vi "Adv_Close_Image.vi"(8 "error in (no error)":errorcluster, 10 "ImageDataSet":refnum<k24>, 11 "LightField Automation in":refnum<class "LightField Automation.lvclass">) -> (0 "error out":errorcluster, 3 "LightField Automation out":refnum<class "LightField Automation.lvclass">)   [LabVIEW 2015, in "LightField Automation.lvclass"]
uses:
  LightField Automation.lvclass
  C:/Program Files/Princeton Instruments/LightField/AddInViews/PrincetonInstruments.LightFieldViewV3.dll
  Program Files/Princeton Instruments/LightField/AddInViews/PrincetonInstruments.LightFieldViewV3.dll
  LightField Automation.lvclass/LightField Automation.ctl
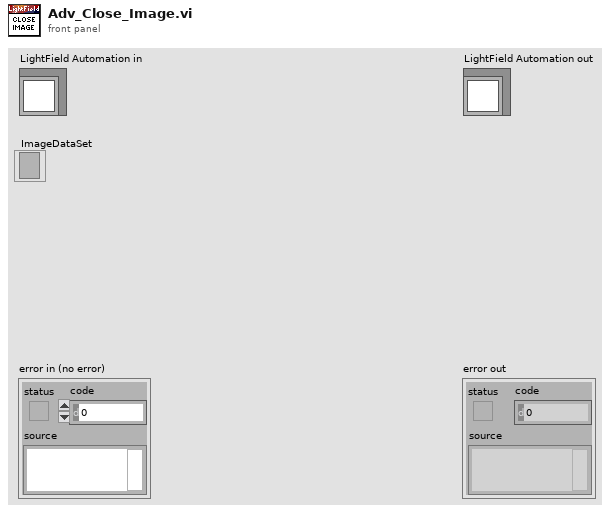
[diagram p1: front panel]
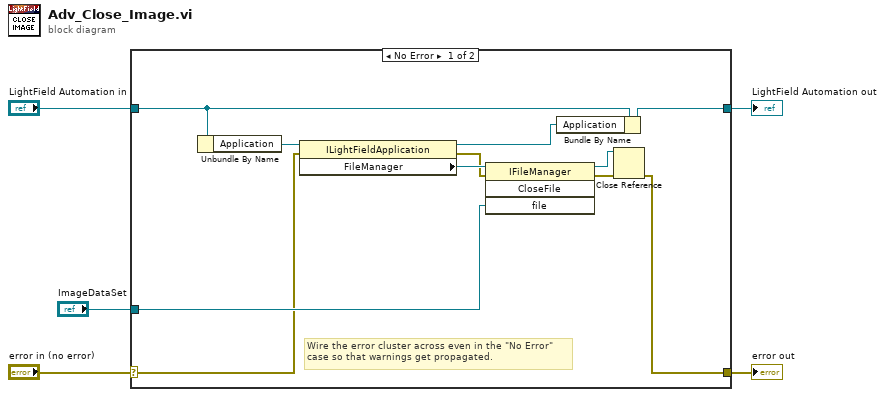
[diagram p0: block diagram]
diagram:
  n1 = case shown="No Error" "error in (no error)" {
    selector: "error in (no error)" -> [w11 w18]
    tunnel: [w6 w18] -> w4
    tunnel: [w8 w17] -> w2
    tunnel: "LightField Automation in" -> [w16 w17]
    tunnel: "ImageDataSet" -> [w13 _]
    frame No Error {
      # "Wire the error cluster across even in the \"No Error\"\ncase so that warnings get propagated."
      n2 = Unbundle By Name(w16) -> ("Application"=w15:refnum<k24>)
      n3 = property class="ILightFieldApplication"(reference=w15, error in=w11) -> (reference out=w7:refnum<k24>, error out=w12:errorcluster, "FileManager"=w14:refnum<k24>)
      n4 = invoke class="IFileManager" method="CloseFile"(reference=w14, error in=w12, "file"=w13) -> (reference out=w9:refnum<k24>, error out=w10:errorcluster)  [unwired: 1 in, 2 out]
      n5 = Bundle By Name(cluster=w16, "Application"=w7) -> (w8:refnum<class "LightField Automation.lvclass">)
      n6 = Close Reference(reference=w9, error in (no error)=w10) -> (error out=w6:errorcluster)
    }
    frame Error {
    }
  }
  "error out" <- w4
  "LightField Automation out" <- w2
